vi "Read DAT File.vi"(8 "error in":errorcluster, 10 "file path (use dialog)":path, 11 "Retrieve and Visualize":refnum<class "Retrieve and Visualize.lvclass">) -> (0 "error out":errorcluster, 3 "Retrieve and Visualize out":refnum<class "Retrieve and Visualize.lvclass">)   [LabVIEW 2016, in "Retrieve and Visualize.lvclass"]
uses:
  Retrieve and Visualize.lvclass
  typedefs/Retrieve and Visualize DAT--Cluster.ctl
  Retrieve and Visualize.lvclass/Retrieve and Visualize.ctl
panel:
  out "timer":dbl
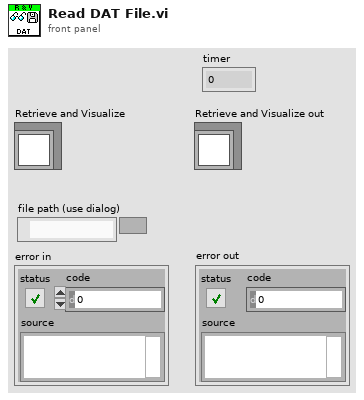
[diagram p1: front panel]
types:
  T1 = typedef "Retrieve and Visualize.lvclass/Retrieve and Visualize DAT--Cluster.ctl" = cluster{"IV":cluster{dbl[], dbl[]}[][][], "IV-2T":cluster{dbl[], dbl[]}[][][], "Vfast":dbl[][], "Vslow":dbl[], "Vslowest":dbl[], "Comments":string, "Scan names":string[]}
  T2 = enum16{"open", "replace", "create", "open or create", "replace or create", "replace or create with confirmation"}
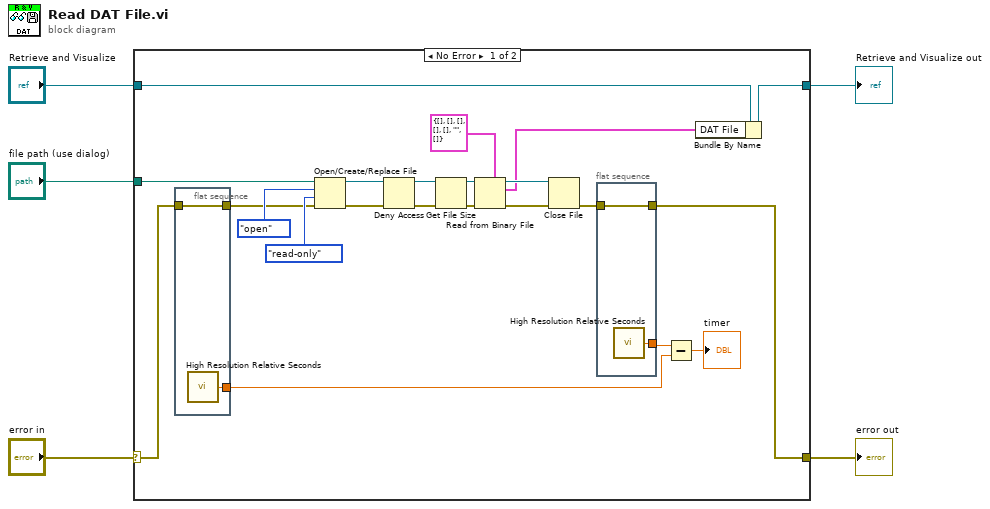
[diagram p0: block diagram]
diagram:
  n1 = case shown="No Error" "error in" {
    selector: "error in" -> [w10 w33]
    tunnel: "file path (use dialog)" -> [w26 _]
    tunnel: [w8 w33] -> w4
    tunnel: "Retrieve and Visualize" -> [w15 w32]
    tunnel: [w14 w32] -> w2
    frame No Error {
      n2 = flat-sequence {
        tunnel: [w29] -> w6
        tunnel: [w28] -> w11
        tunnel: w10 -> [w28]
        frame #0 {
          n3 = call <vilib>:"High Resolution Relative Seconds.vi"() -> ("relative seconds"=w29:dbl)
        }
      }
      n4 = Open/Create/Replace File(file path (use dialog)=w26, error in=w11, operation (0:open)=T2."open", access (0:read/write)=enum16{"read/write", "read-only", "write-only"}."read-only") -> (refnum out=w22:refnum<file>, error out=w21:errorcluster)  [unwired: 2 in, 1 out]
      n5 = Deny Access(4:w21, 7:w22) -> (0:w23:errorcluster, 3:w24:refnum<file>)  [unwired: 1 in]
      n6 = Get File Size(file=w24, error in=w23) -> (refnum out=w16:refnum<file>, 0:w19:errorcluster)  [unwired: 1 out]
      n7 = Read from Binary File(5:T1 {"IV"=[], "IV-2T"=[], "Vfast"=[], "Vslow"=[], "Vslowest"=[], "Comments"="", "Scan names"=[]} ("output cluster"), 8:w19, 11:w16) -> (0:w18:errorcluster, 2:w12:T1, 3:w17:refnum<file>)  [unwired: 3 in, 1 out]
      n8 = Close File(refnum=w17, error in=w18) -> (error out=w9:errorcluster)  [unwired: 1 out]
      n9 = flat-sequence {
        tunnel: [w31] -> w27
        tunnel: w9 -> [w30]
        tunnel: [w30] -> w8
        frame #0 {
          n10 = call <vilib>:"High Resolution Relative Seconds.vi"() -> ("relative seconds"=w31:dbl)
        }
      }
      n11 = Subtract(x=w27, y=w6) -> (x-y=→"timer":dbl)
      n12 = Bundle By Name(cluster=w15, "DAT File"=w12) -> (w14:refnum<class "Retrieve and Visualize.lvclass">)
    }
    frame Error {
    }
  }
  "error out" <- w4
  "Retrieve and Visualize out" <- w2
